vi "GetInputFrequency.vi"(0 "Signal Type Select":u16(ring) items=["1Mhz", "1MHz MONITOR PLUG", "DSMP", "DSMP MONITOR PLUG", "RP", "RP MONITOR PLUG", "MP", "MP MONITOR PLUG", "EEP 1.2 Sec", "EEP MONITOR PLUG", "SMP DIFF", "SMP MONITOR PLUG", "SMP Open Collector"], 1 "Connection ID IN":refnum<k5>, 2 "ERROR IN":errorcluster) -> (5 "Success":bool, 6 "Result":string, 7 "DECIMAL":u32, 8 "ERROR OUT":errorcluster)   [LabVIEW 2013]
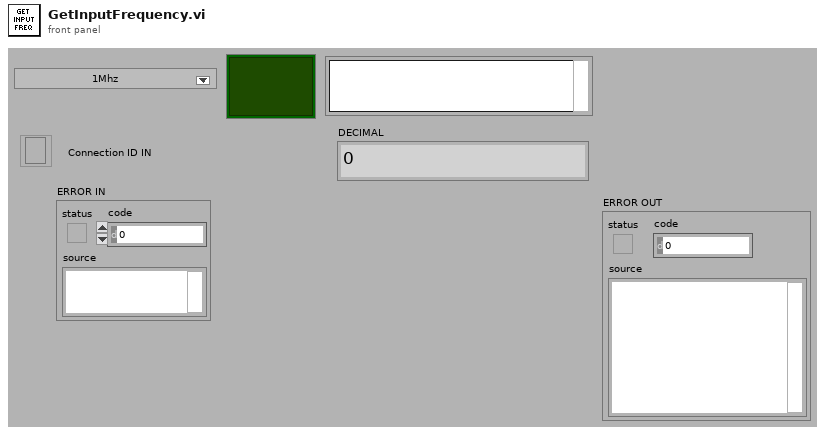
[diagram p1: front panel]
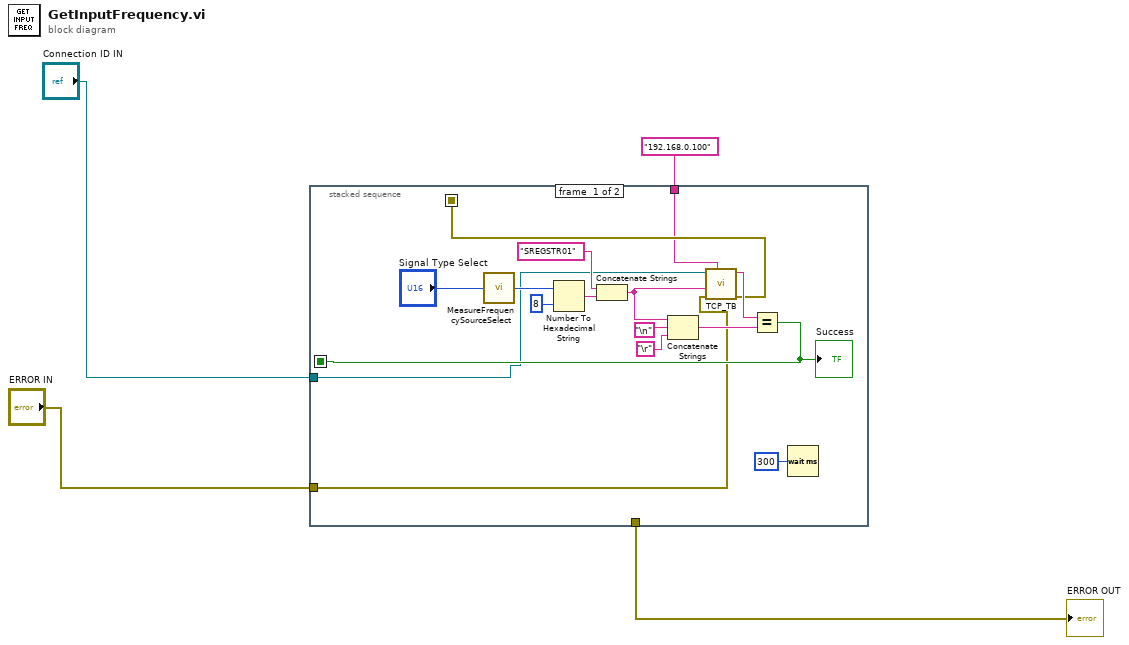
[diagram p0: block diagram]
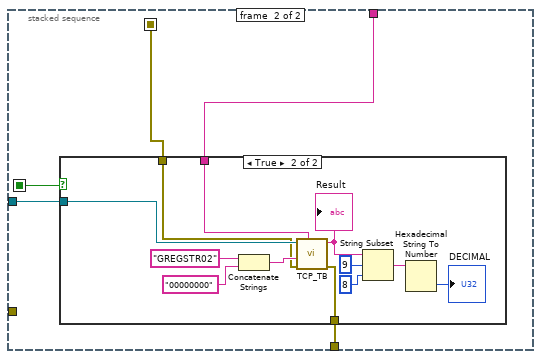
[diagram p2: hidden frame]
diagram:
  n1 = stacked-sequence {
    seq-local: [w11 _] -> [_ w24]
    seq-local: [w9 _] -> [_ w22]
    tunnel: "192.168.0.100" ("IP ADDRESS") -> [w7 w25]
    tunnel: "ERROR IN" -> [w10 _]
    tunnel: "Connection ID IN" -> [w6 w23]
    tunnel: [_ w21] -> w2
    frame #0 {
      n2 = call "MeasureFrequencySourceSelect.vi"("Signal Type Select"="Signal Type Select") -> ("Numeric"=w18:i32)
      n3 = Number To Hexadecimal String(1:i16 8 ("width (-)"), 2:w18) -> (0:w19:string)
      n4 = Concatenate Strings("SREGSTR01" ("COMMAND"), w19) -> (w16:string)
      n5 = Concatenate Strings(w16, "\n", "\r") -> (w15:string)
      n6 = call "TCP_TB.vi"("IP ADDRESS"=w7, "error in (no error)"=w10, "COMMAND"=w16, "Connection ID IN"=w6) -> ("error out"=w9:errorcluster, "Their Response:"=w13:string)  [unwired: 2 in, 1 out]
      n7 = Equal?(x=w13, y=w15) -> (x = y?=w11:bool)
      "Success" <- w11
      n8 = Wait (ms)(milliseconds to wait=u32 300) -> ()  [unwired: 1 out]
    }
    frame #1 {
      n9 = case shown="True" w24 {
        tunnel: w25 -> [_ w30]
        tunnel: w23 -> [_ w29]
        tunnel: w22 -> [w26 w28]
        tunnel: [w26 w27] -> w21
        frame False {
        }
        frame True {
          n10 = Concatenate Strings("GREGSTR02" ("COMMAND"), "00000000" ("string")) -> (w37:string)
          n11 = call "TCP_TB.vi"("IP ADDRESS"=w30, "error in (no error)"=w28, "COMMAND"=w37, "Connection ID IN"=w29) -> ("error out"=w27:errorcluster, "Their Response:"=w35:string)  [unwired: 2 in, 1 out]
          "Result" <- w35
          n12 = String Subset(string=w35, offset (0)=9, length (rest)=8 ("length (rest)")) -> (substring=w32:string)
          n13 = Hexadecimal String To Number(string=w32) -> (number=→"DECIMAL":u32)  [unwired: 2 in, 1 out]
        }
      }
    }
  }
  "ERROR OUT" <- w2
